vi "Read Constant.vi"(8 "error in (no error)":errorcluster, 11 "ArgumentConfig in":refnum<class "ArgumentConfig.lvclass">) -> (0 "error out":errorcluster, 2 "Constant":string, 3 "ArgumentConfig out":refnum<class "ArgumentConfig.lvclass">)   [LabVIEW 2022 SP3, in "ArgumentParser.lvlib" / "ArgumentConfig.lvclass"]
uses:
  ArgumentConfig.lvclass
  ArgumentConfig.lvclass/ArgumentConfig.ctl
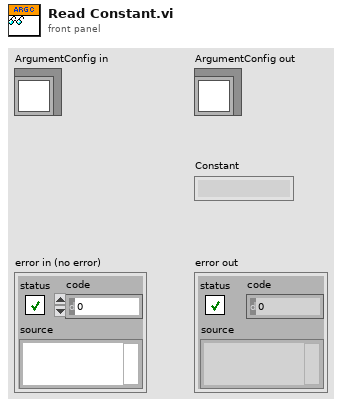
[diagram p1: front panel]
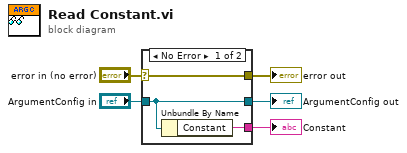
[diagram p0: block diagram]
diagram:
  n1 = case shown="No Error" "error in (no error)" {
    selector: "error in (no error)" -> [w8 w9]
    tunnel: [w8 w9] -> w4
    tunnel: [w7 w10] -> w2
    tunnel: "ArgumentConfig in" -> [w7 w10]
    tunnel: [w6 _] -> w1
    frame No Error {
      n2 = Unbundle By Name(w7) -> ("Constant"=w6:string)
    }
    frame Error {
    }
  }
  "error out" <- w4
  "ArgumentConfig out" <- w2
  "Constant" <- w1
